vi "Excel input(SubVI).vi"(8 "error in (no error)":errorcluster, 11 "The Path to save excel":path=path "E:/程序完善/油菜/side_features") -> (0 "error out":errorcluster, 3 "Cluster":T1)   [LabVIEW 2015]
uses:
  <vilib>/Utility/NIReport.llb/NI_report.lvclass
  <vilib>/addons/_office/_exclsub.llb/font.ctl
  <vilib>/addons/_office/NI_ReportGenerationToolkit.lvlib
  <vilib>/Utility/NIReport.llb/Excel/NI_Excel.lvclass
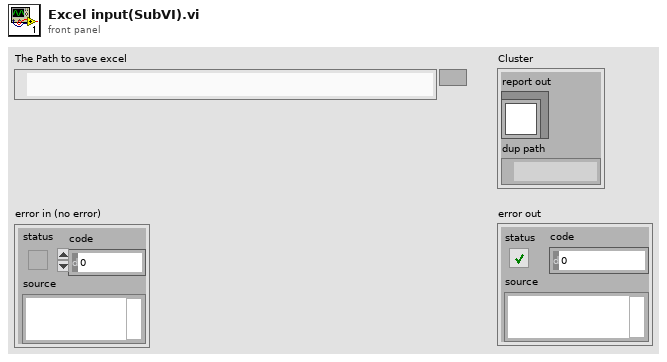
[diagram p1: front panel]
types:
  T1 = cluster{"report out":refnum<class "NI_report.lvclass">, "dup path":path}
  T2 = enum16{"maximized", "minimized", "normal", "no change"}
  T3 = typedef "NI_ReportGenerationToolkit.lvlib/font.ctl" = cluster{"font name":string, "font size":dbl, "bold":u16, "italic":u16, "underline":u16, "strike through":u16, "font color":u32}
  T4 = enum16{"Standard Report", "HTML", "Word", "Excel"}
diagram:
  w408 = T3 {"font name"="", "font size"=13.0, "bold"=0, "italic"=0, "underline"=0, "strike through"=0, "font color"=16777216} ("font")
  w106 = 0 ("column")
  n1 = call <vilib>:"New Report.vi"("window state (normal)"=T2."normal", "report type"=T4."Excel", "error in (no error)"="error in (no error)") -> ("report out"=w10:refnum<class "NI_report.lvclass">, "error out"=w7:errorcluster)  [unwired: 3 in, 8 out]
  n2 = call <vilib>:"Excel Easy Title.vi"("report in"=w10, "title"="Side Features", "start (0, 0)"=cluster{"row":i32, "column":i32} {"row"=0, "column"=0}, "font"=T3 {"font name"="", "font size"=16.0, "bold"=1, "italic"=2, "underline"=2, "strike through"=2, "font color"=0}, "error in (no error)"=w7) -> ("report out"=w107:refnum<class "NI_report.lvclass">, "error out"=w110:errorcluster)  [unwired: 1 in, 8 out]
  n3 = Bundle("row"=1, "column"=w106) -> (w109:cluster{"row":i32, "column":i32})  [unwired: 1 out]
  n4 = Increment(x=w106) -> (x+1=w45:i32)
  n5 = call <vilib>:"Excel Easy Text.vi"("report in"=w107, "border? (F)"=FALSE, "font"=w408, "text"="Serial number", "start (-1, -1)"=w109, "error in (no error)"=w110) -> ("report out"=w56:refnum<class "NI_report.lvclass">, "error out"=w43:errorcluster)  [unwired: 2 in, 6 out]
  n6 = Bundle("row"=1, w45) -> (w60:cluster{"row":i32, i32})  [unwired: 1 out]
  n7 = Increment(x=w45) -> (x+1=w44:i32)
  n8 = call <vilib>:"Excel Easy Text.vi"("report in"=w56, "border? (F)"=FALSE, "font"=w408, "text"="M_TEX_SV", "start (-1, -1)"=w60, "error in (no error)"=w43) -> ("report out"=w47:refnum<class "NI_report.lvclass">, "error out"=w42:errorcluster)  [unwired: 2 in, 6 out]
  n9 = Bundle("row"=1, w44) -> (w52:cluster{"row":i32, i32})  [unwired: 1 out]
  n10 = Increment(x=w44) -> (x+1=w20:i32)
  n11 = call <vilib>:"Excel Easy Text.vi"("report in"=w47, "border? (F)"=FALSE, "font"=w408, "text"="SE_TEX_SV", "start (-1, -1)"=w52, "error in (no error)"=w42) -> ("report out"=w46:refnum<class "NI_report.lvclass">, "error out"=w41:errorcluster)  [unwired: 2 in, 6 out]
  n12 = Bundle("row"=1, w20) -> (w51:cluster{"row":i32, i32})  [unwired: 1 out]
  n13 = Increment(x=w20) -> (x+1=w26:i32)
  n14 = call <vilib>:"Excel Easy Text.vi"("report in"=w46, "border? (F)"=FALSE, "font"=w408, "text"="S_TEX_SV", "start (-1, -1)"=w51, "error in (no error)"=w41) -> ("report out"=w21:refnum<class "NI_report.lvclass">, "error out"=w22:errorcluster)  [unwired: 2 in, 6 out]
  n15 = Bundle("row"=1, w26) -> (w40:cluster{"row":i32, i32})  [unwired: 1 out]
  n16 = Increment(x=w26) -> (x+1=w25:i32)
  n17 = call <vilib>:"Excel Easy Text.vi"("report in"=w21, "border? (F)"=FALSE, "font"=w408, "text"="MU3_TEX_SV", "start (-1, -1)"=w40, "error in (no error)"=w22) -> ("report out"=w28:refnum<class "NI_report.lvclass">, "error out"=w24:errorcluster)  [unwired: 2 in, 6 out]
  n18 = Bundle("row"=1, w25) -> (w33:cluster{"row":i32, i32})  [unwired: 1 out]
  n19 = Increment(x=w25) -> (x+1=w13:i32)
  n20 = call <vilib>:"Excel Easy Text.vi"("report in"=w28, "border? (F)"=FALSE, "font"=w408, "text"="U_TEX_SV", "start (-1, -1)"=w33, "error in (no error)"=w24) -> ("report out"=w27:refnum<class "NI_report.lvclass">, "error out"=w23:errorcluster)  [unwired: 2 in, 6 out]
  n21 = Bundle("row"=1, w13) -> (w32:cluster{"row":i32, i32})  [unwired: 1 out]
  n22 = Increment(x=w13) -> (x+1=w75:i32)
  n23 = call <vilib>:"Excel Easy Text.vi"("report in"=w27, "border? (F)"=FALSE, "font"=w408, "text"="E_TEX_SV", "start (-1, -1)"=w32, "error in (no error)"=w23) -> ("report out"=w15:refnum<class "NI_report.lvclass">, "error out"=w14:errorcluster)  [unwired: 2 in, 6 out]
  n24 = Bundle("row"=1, w75) -> (w16:cluster{"row":i32, i32})  [unwired: 1 out]
  n25 = Increment(x=w75) -> (x+1=w78:i32)
  n26 = call <vilib>:"Excel Easy Text.vi"("report in"=w15, "border? (F)"=FALSE, "font"=w408, "text"="TPA_SV", "start (-1, -1)"=w16, "error in (no error)"=w14) -> ("report out"=w73:refnum<class "NI_report.lvclass">, "error out"=w74:errorcluster)  [unwired: 2 in, 6 out]
  n27 = Bundle("row"=1, w78) -> (w69:cluster{"row":i32, i32})  [unwired: 1 out]
  n28 = Increment(x=w78) -> (x+1=w81:i32)
  n29 = call <vilib>:"Excel Easy Text.vi"("report in"=w73, "border? (F)"=FALSE, "font"=w408, "text"="H_SV", "start (-1, -1)"=w69, "error in (no error)"=w74) -> ("report out"=w76:refnum<class "NI_report.lvclass">, "error out"=w77:errorcluster)  [unwired: 2 in, 6 out]
  n30 = Bundle("row"=1, w81) -> (w61:cluster{"row":i32, i32})  [unwired: 1 out]
  n31 = Increment(x=w81) -> (x+1=w88:i32)
  n32 = call <vilib>:"Excel Easy Text.vi"("report in"=w76, "border? (F)"=FALSE, "font"=w408, "text"="W_SV", "start (-1, -1)"=w61, "error in (no error)"=w77) -> ("report out"=w79:refnum<class "NI_report.lvclass">, "error out"=w80:errorcluster)  [unwired: 2 in, 6 out]
  n33 = Bundle("row"=1, w88) -> (w65:cluster{"row":i32, i32})  [unwired: 1 out]
  n34 = Increment(x=w88) -> (x+1=w95:i32)
  n35 = call <vilib>:"Excel Easy Text.vi"("report in"=w79, "border? (F)"=FALSE, "font"=w408, "text"="HWR_SV", "start (-1, -1)"=w65, "error in (no error)"=w80) -> ("report out"=w86:refnum<class "NI_report.lvclass">, "error out"=w87:errorcluster)  [unwired: 2 in, 6 out]
  n36 = Bundle("row"=1, w95) -> (w82:cluster{"row":i32, i32})  [unwired: 1 out]
  n37 = Increment(x=w95) -> (x+1=w102:i32)
  n38 = call <vilib>:"Excel Easy Text.vi"("report in"=w86, "border? (F)"=FALSE, "font"=w408, "text"="FDNIC_SV", "start (-1, -1)"=w82, "error in (no error)"=w87) -> ("report out"=w93:refnum<class "NI_report.lvclass">, "error out"=w94:errorcluster)  [unwired: 2 in, 6 out]
  n39 = Bundle("row"=1, w102) -> (w89:cluster{"row":i32, i32})  [unwired: 1 out]
  n40 = Increment(x=w102) -> (x+1=w104:i32)
  n41 = call <vilib>:"Excel Easy Text.vi"("report in"=w93, "border? (F)"=FALSE, "font"=w408, "text"="FDIC_SV", "start (-1, -1)"=w89, "error in (no error)"=w94) -> ("report out"=w100:refnum<class "NI_report.lvclass">, "error out"=w101:errorcluster)  [unwired: 2 in, 6 out]
  n42 = Bundle("row"=1, w104) -> (w96:cluster{"row":i32, i32})  [unwired: 1 out]
  n43 = Increment(x=w104) -> (x+1=w151:i32)
  n44 = call <vilib>:"Excel Easy Text.vi"("report in"=w100, "border? (F)"=FALSE, "font"=w408, "text"="R_SV", "start (-1, -1)"=w96, "error in (no error)"=w101) -> ("report out"=w150:refnum<class "NI_report.lvclass">, "error out"=w152:errorcluster)  [unwired: 2 in, 6 out]
  n45 = Bundle("row"=1, w151) -> (w149:cluster{"row":i32, i32})  [unwired: 1 out]
  n46 = Increment(x=w151) -> (x+1=w125:i32)
  n47 = call <vilib>:"Excel Easy Text.vi"("report in"=w150, "border? (F)"=FALSE, "font"=w408, "text"="PAR_SV", "start (-1, -1)"=w149, "error in (no error)"=w152) -> ("report out"=w121:refnum<class "NI_report.lvclass">, "error out"=w122:errorcluster)  [unwired: 2 in, 6 out]
  n48 = Bundle("row"=1, w125) -> (w111:cluster{"row":i32, i32})  [unwired: 1 out]
  n49 = Increment(x=w125) -> (x+1=w132:i32)
  n50 = call <vilib>:"Excel Easy Text.vi"("report in"=w121, "border? (F)"=FALSE, "font"=w408, "text"="HA_SV", "start (-1, -1)"=w111, "error in (no error)"=w122) -> ("report out"=w123:refnum<class "NI_report.lvclass">, "error out"=w124:errorcluster)  [unwired: 2 in, 6 out]
  n51 = Bundle("row"=1, w132) -> (w115:cluster{"row":i32, i32})  [unwired: 1 out]
  n52 = Increment(x=w132) -> (x+1=w139:i32)
  n53 = call <vilib>:"Excel Easy Text.vi"("report in"=w123, "border? (F)"=FALSE, "font"=w408, "text"="AC_SV", "start (-1, -1)"=w115, "error in (no error)"=w124) -> ("report out"=w130:refnum<class "NI_report.lvclass">, "error out"=w131:errorcluster)  [unwired: 2 in, 6 out]
  n54 = Bundle("row"=1, w139) -> (w126:cluster{"row":i32, i32})  [unwired: 1 out]
  n55 = Increment(x=w139) -> (x+1=w146:i32)
  n56 = call <vilib>:"Excel Easy Text.vi"("report in"=w130, "border? (F)"=FALSE, "font"=w408, "text"="M_TEX_SV_FL", "start (-1, -1)"=w126, "error in (no error)"=w131) -> ("report out"=w137:refnum<class "NI_report.lvclass">, "error out"=w138:errorcluster)  [unwired: 2 in, 6 out]
  n57 = Bundle("row"=1, w146) -> (w133:cluster{"row":i32, i32})  [unwired: 1 out]
  n58 = Increment(x=w146) -> (x+1=w148:i32)
  n59 = call <vilib>:"Excel Easy Text.vi"("report in"=w137, "border? (F)"=FALSE, "font"=w408, "text"="SE_TEX_SV_FL", "start (-1, -1)"=w133, "error in (no error)"=w138) -> ("report out"=w144:refnum<class "NI_report.lvclass">, "error out"=w145:errorcluster)  [unwired: 2 in, 6 out]
  n60 = Bundle("row"=1, w148) -> (w140:cluster{"row":i32, i32})  [unwired: 1 out]
  n61 = Increment(x=w148) -> (x+1=w219:i32)
  n62 = call <vilib>:"Excel Easy Text.vi"("report in"=w144, "border? (F)"=FALSE, "font"=w408, "text"="S_TEX_SV_FL", "start (-1, -1)"=w140, "error in (no error)"=w145) -> ("report out"=w221:refnum<class "NI_report.lvclass">, "error out"=w222:errorcluster)  [unwired: 2 in, 6 out]
  n63 = Bundle("row"=1, w219) -> (w220:cluster{"row":i32, i32})  [unwired: 1 out]
  n64 = Increment(x=w219) -> (x+1=w167:i32)
  n65 = call <vilib>:"Excel Easy Text.vi"("report in"=w221, "border? (F)"=FALSE, "font"=w408, "text"="MU3_TEX_SV_FL", "start (-1, -1)"=w220, "error in (no error)"=w222) -> ("report out"=w159:refnum<class "NI_report.lvclass">, "error out"=w160:errorcluster)  [unwired: 2 in, 6 out]
  n66 = Bundle("row"=1, w167) -> (w155:cluster{"row":i32, i32})  [unwired: 1 out]
  n67 = Increment(x=w167) -> (x+1=w174:i32)
  n68 = call <vilib>:"Excel Easy Text.vi"("report in"=w159, "border? (F)"=FALSE, "font"=w408, "text"="U_TEX_SV_FL", "start (-1, -1)"=w155, "error in (no error)"=w160) -> ("report out"=w165:refnum<class "NI_report.lvclass">, "error out"=w166:errorcluster)  [unwired: 2 in, 6 out]
  n69 = Bundle("row"=1, w174) -> (w161:cluster{"row":i32, i32})  [unwired: 1 out]
  n70 = Increment(x=w174) -> (x+1=w176:i32)
  n71 = call <vilib>:"Excel Easy Text.vi"("report in"=w165, "border? (F)"=FALSE, "font"=w408, "text"="E_TEX_SV_FL", "start (-1, -1)"=w161, "error in (no error)"=w166) -> ("report out"=w172:refnum<class "NI_report.lvclass">, "error out"=w173:errorcluster)  [unwired: 2 in, 6 out]
  n72 = Bundle("row"=1, w176) -> (w168:cluster{"row":i32, i32})  [unwired: 1 out]
  n73 = Increment(x=w176) -> (x+1=w217:i32)
  n74 = call <vilib>:"Excel Easy Text.vi"("report in"=w172, "border? (F)"=FALSE, "font"=w408, "text"="YPA_SV_FL", "start (-1, -1)"=w168, "error in (no error)"=w173) -> ("report out"=w216:refnum<class "NI_report.lvclass">, "error out"=w218:errorcluster)  [unwired: 2 in, 6 out]
  n75 = Bundle("row"=1, w217) -> (w215:cluster{"row":i32, i32})  [unwired: 1 out]
  n76 = Increment(x=w217) -> (x+1=w191:i32)
  n77 = call <vilib>:"Excel Easy Text.vi"("report in"=w216, "border? (F)"=FALSE, "font"=w408, "text"="H_SV_FL", "start (-1, -1)"=w215, "error in (no error)"=w218) -> ("report out"=w187:refnum<class "NI_report.lvclass">, "error out"=w188:errorcluster)  [unwired: 2 in, 6 out]
  n78 = Bundle("row"=1, w191) -> (w177:cluster{"row":i32, i32})  [unwired: 1 out]
  n79 = Increment(x=w191) -> (x+1=w198:i32)
  n80 = call <vilib>:"Excel Easy Text.vi"("report in"=w187, "border? (F)"=FALSE, "font"=w408, "text"="W_SV_FL", "start (-1, -1)"=w177, "error in (no error)"=w188) -> ("report out"=w189:refnum<class "NI_report.lvclass">, "error out"=w190:errorcluster)  [unwired: 2 in, 6 out]
  n81 = Bundle("row"=1, w198) -> (w181:cluster{"row":i32, i32})  [unwired: 1 out]
  n82 = Increment(x=w198) -> (x+1=w205:i32)
  n83 = call <vilib>:"Excel Easy Text.vi"("report in"=w189, "border? (F)"=FALSE, "font"=w408, "text"="HWR_SV_FL", "start (-1, -1)"=w181, "error in (no error)"=w190) -> ("report out"=w196:refnum<class "NI_report.lvclass">, "error out"=w197:errorcluster)  [unwired: 2 in, 6 out]
  n84 = Bundle("row"=1, w205) -> (w192:cluster{"row":i32, i32})  [unwired: 1 out]
  n85 = Increment(x=w205) -> (x+1=w212:i32)
  n86 = call <vilib>:"Excel Easy Text.vi"("report in"=w196, "border? (F)"=FALSE, "font"=w408, "text"="FDNIC_SV_FL", "start (-1, -1)"=w192, "error in (no error)"=w197) -> ("report out"=w203:refnum<class "NI_report.lvclass">, "error out"=w204:errorcluster)  [unwired: 2 in, 6 out]
  n87 = Bundle("row"=1, w212) -> (w199:cluster{"row":i32, i32})  [unwired: 1 out]
  n88 = Increment(x=w212) -> (x+1=w214:i32)
  n89 = call <vilib>:"Excel Easy Text.vi"("report in"=w203, "border? (F)"=FALSE, "font"=w408, "text"="FDIC_SV_FL", "start (-1, -1)"=w199, "error in (no error)"=w204) -> ("report out"=w210:refnum<class "NI_report.lvclass">, "error out"=w211:errorcluster)  [unwired: 2 in, 6 out]
  n90 = Bundle("row"=1, w214) -> (w206:cluster{"row":i32, i32})  [unwired: 1 out]
  n91 = Increment(x=w214) -> (x+1=w338:i32)
  n92 = call <vilib>:"Excel Easy Text.vi"("report in"=w210, "border? (F)"=FALSE, "font"=w408, "text"="R_SV_FL", "start (-1, -1)"=w206, "error in (no error)"=w211) -> ("report out"=w339:refnum<class "NI_report.lvclass">, "error out"=w340:errorcluster)  [unwired: 2 in, 6 out]
  n93 = Bundle("row"=1, w338) -> (w341:cluster{"row":i32, i32})  [unwired: 1 out]
  n94 = Increment(x=w338) -> (x+1=w266:i32)
  n95 = call <vilib>:"Excel Easy Text.vi"("report in"=w339, "border? (F)"=FALSE, "font"=w408, "text"="PAR_SV_FL", "start (-1, -1)"=w341, "error in (no error)"=w340) -> ("report out"=w265:refnum<class "NI_report.lvclass">, "error out"=w267:errorcluster)  [unwired: 2 in, 6 out]
  n96 = Bundle("row"=1, w266) -> (w264:cluster{"row":i32, i32})  [unwired: 1 out]
  n97 = Increment(x=w266) -> (x+1=w240:i32)
  n98 = call <vilib>:"Excel Easy Text.vi"("report in"=w265, "border? (F)"=FALSE, "font"=w408, "text"="HA_SV_FL", "start (-1, -1)"=w264, "error in (no error)"=w267) -> ("report out"=w236:refnum<class "NI_report.lvclass">, "error out"=w237:errorcluster)  [unwired: 2 in, 6 out]
  n99 = Bundle("row"=1, w240) -> (w226:cluster{"row":i32, i32})  [unwired: 1 out]
  n100 = Increment(x=w240) -> (x+1=w247:i32)
  n101 = call <vilib>:"Excel Easy Text.vi"("report in"=w236, "border? (F)"=FALSE, "font"=w408, "text"="AC_SV_FL", "start (-1, -1)"=w226, "error in (no error)"=w237) -> ("report out"=w238:refnum<class "NI_report.lvclass">, "error out"=w239:errorcluster)  [unwired: 2 in, 6 out]
  n102 = Bundle("row"=1, w247) -> (w230:cluster{"row":i32, i32})  [unwired: 1 out]
  n103 = Increment(x=w247) -> (x+1=w254:i32)
  n104 = call <vilib>:"Excel Easy Text.vi"("report in"=w238, "border? (F)"=FALSE, "font"=w408, "text"="FN_SV", "start (-1, -1)"=w230, "error in (no error)"=w239) -> ("report out"=w245:refnum<class "NI_report.lvclass">, "error out"=w246:errorcluster)  [unwired: 2 in, 6 out]
  n105 = Bundle("row"=1, w254) -> (w241:cluster{"row":i32, i32})  [unwired: 1 out]
  n106 = Increment(x=w254) -> (x+1=w261:i32)
  n107 = call <vilib>:"Excel Easy Text.vi"("report in"=w245, "border? (F)"=FALSE, "font"=w408, "text"="GPA_SV", "start (-1, -1)"=w241, "error in (no error)"=w246) -> ("report out"=w252:refnum<class "NI_report.lvclass">, "error out"=w253:errorcluster)  [unwired: 2 in, 6 out]
  n108 = Bundle("row"=1, w261) -> (w248:cluster{"row":i32, i32})  [unwired: 1 out]
  n109 = Increment(x=w261) -> (x+1=w263:i32)
  n110 = call <vilib>:"Excel Easy Text.vi"("report in"=w252, "border? (F)"=FALSE, "font"=w408, "text"="GPAR_SV", "start (-1, -1)"=w248, "error in (no error)"=w253) -> ("report out"=w259:refnum<class "NI_report.lvclass">, "error out"=w260:errorcluster)  [unwired: 2 in, 6 out]
  n111 = Bundle("row"=1, w263) -> (w255:cluster{"row":i32, i32})  [unwired: 1 out]
  n112 = Increment(x=w263) -> (x+1=w334:i32)
  n113 = call <vilib>:"Excel Easy Text.vi"("report in"=w259, "border? (F)"=FALSE, "font"=w408, "text"="YPAR_SV", "start (-1, -1)"=w255, "error in (no error)"=w260) -> ("report out"=w336:refnum<class "NI_report.lvclass">, "error out"=w337:errorcluster)  [unwired: 2 in, 6 out]
  n114 = Bundle("row"=1, w334) -> (w335:cluster{"row":i32, i32})  [unwired: 1 out]
  n115 = Increment(x=w334) -> (x+1=w282:i32)
  n116 = call <vilib>:"Excel Easy Text.vi"("report in"=w336, "border? (F)"=FALSE, "font"=w408, "text"="PC1_SV", "start (-1, -1)"=w335, "error in (no error)"=w337) -> ("report out"=w274:refnum<class "NI_report.lvclass">, "error out"=w275:errorcluster)  [unwired: 2 in, 6 out]
  n117 = Bundle("row"=1, w282) -> (w270:cluster{"row":i32, i32})  [unwired: 1 out]
  n118 = Increment(x=w282) -> (x+1=w289:i32)
  n119 = call <vilib>:"Excel Easy Text.vi"("report in"=w274, "border? (F)"=FALSE, "font"=w408, "text"="PC2_SV", "start (-1, -1)"=w270, "error in (no error)"=w275) -> ("report out"=w280:refnum<class "NI_report.lvclass">, "error out"=w281:errorcluster)  [unwired: 2 in, 6 out]
  n120 = Bundle("row"=1, w289) -> (w276:cluster{"row":i32, i32})  [unwired: 1 out]
  n121 = Increment(x=w289) -> (x+1=w291:i32)
  n122 = call <vilib>:"Excel Easy Text.vi"("report in"=w280, "border? (F)"=FALSE, "font"=w408, "text"="PC3_SV", "start (-1, -1)"=w276, "error in (no error)"=w281) -> ("report out"=w287:refnum<class "NI_report.lvclass">, "error out"=w288:errorcluster)  [unwired: 2 in, 6 out]
  n123 = Bundle("row"=1, w291) -> (w283:cluster{"row":i32, i32})  [unwired: 1 out]
  n124 = Increment(x=w291) -> (x+1=w332:i32)
  n125 = call <vilib>:"Excel Easy Text.vi"("report in"=w287, "border? (F)"=FALSE, "font"=w408, "text"="PC4_SV", "start (-1, -1)"=w283, "error in (no error)"=w288) -> ("report out"=w331:refnum<class "NI_report.lvclass">, "error out"=w333:errorcluster)  [unwired: 2 in, 6 out]
  n126 = Bundle("row"=1, w332) -> (w330:cluster{"row":i32, i32})  [unwired: 1 out]
  n127 = Increment(x=w332) -> (x+1=w306:i32)
  n128 = call <vilib>:"Excel Easy Text.vi"("report in"=w331, "border? (F)"=FALSE, "font"=w408, "text"="PC5_SV", "start (-1, -1)"=w330, "error in (no error)"=w333) -> ("report out"=w302:refnum<class "NI_report.lvclass">, "error out"=w303:errorcluster)  [unwired: 2 in, 6 out]
  n129 = Bundle("row"=1, w306) -> (w292:cluster{"row":i32, i32})  [unwired: 1 out]
  n130 = Increment(x=w306) -> (x+1=w313:i32)
  n131 = call <vilib>:"Excel Easy Text.vi"("report in"=w302, "border? (F)"=FALSE, "font"=w408, "text"="PC6_SV", "start (-1, -1)"=w292, "error in (no error)"=w303) -> ("report out"=w304:refnum<class "NI_report.lvclass">, "error out"=w305:errorcluster)  [unwired: 2 in, 6 out]
  n132 = Bundle("row"=1, w313) -> (w296:cluster{"row":i32, i32})  [unwired: 1 out]
  n133 = Increment(x=w313) -> (x+1=w320:i32)
  n134 = call <vilib>:"Excel Easy Text.vi"("report in"=w304, "border? (F)"=FALSE, "font"=w408, "text"="F1", "start (-1, -1)"=w296, "error in (no error)"=w305) -> ("report out"=w311:refnum<class "NI_report.lvclass">, "error out"=w312:errorcluster)  [unwired: 2 in, 6 out]
  n135 = Bundle("row"=1, w320) -> (w307:cluster{"row":i32, i32})  [unwired: 1 out]
  n136 = Increment(x=w320) -> (x+1=w327:i32)
  n137 = call <vilib>:"Excel Easy Text.vi"("report in"=w311, "border? (F)"=FALSE, "font"=w408, "text"="F2", "start (-1, -1)"=w307, "error in (no error)"=w312) -> ("report out"=w318:refnum<class "NI_report.lvclass">, "error out"=w319:errorcluster)  [unwired: 2 in, 6 out]
  n138 = Bundle("row"=1, w327) -> (w314:cluster{"row":i32, i32})  [unwired: 1 out]
  n139 = Increment(x=w327) -> (x+1=w329:i32)
  n140 = call <vilib>:"Excel Easy Text.vi"("report in"=w318, "border? (F)"=FALSE, "font"=w408, "text"="F3", "start (-1, -1)"=w314, "error in (no error)"=w319) -> ("report out"=w325:refnum<class "NI_report.lvclass">, "error out"=w326:errorcluster)  [unwired: 2 in, 6 out]
  n141 = Bundle("row"=1, w329) -> (w321:cluster{"row":i32, i32})  [unwired: 1 out]
  n142 = Increment(x=w329) -> (x+1=w411:i32)
  n143 = call <vilib>:"Excel Easy Text.vi"("report in"=w325, "border? (F)"=FALSE, "font"=w408, "text"="F4", "start (-1, -1)"=w321, "error in (no error)"=w326) -> ("report out"=w410:refnum<class "NI_report.lvclass">, "error out"=w407:errorcluster)  [unwired: 2 in, 6 out]
  n144 = Bundle("row"=1, w411) -> (w409:cluster{"row":i32, i32})  [unwired: 1 out]
  n145 = Increment(x=w411) -> (x+1=w351:i32)
  n146 = call <vilib>:"Excel Easy Text.vi"("report in"=w410, "border? (F)"=FALSE, "font"=w408, "text"="F5", "start (-1, -1)"=w409, "error in (no error)"=w407) -> ("report out"=w348:refnum<class "NI_report.lvclass">, "error out"=w349:errorcluster)  [unwired: 2 in, 6 out]
  n147 = Bundle("row"=1, w351) -> (w344:cluster{"row":i32, i32})  [unwired: 1 out]
  n148 = Increment(x=w351) -> (x+1=w403:i32)
  n149 = call <vilib>:"Excel Easy Text.vi"("report in"=w348, "border? (F)"=FALSE, "font"=w408, "text"="F6", "start (-1, -1)"=w344, "error in (no error)"=w349) -> ("report out"=w405:refnum<class "NI_report.lvclass">, "error out"=w406:errorcluster)  [unwired: 2 in, 6 out]
  n150 = Bundle("row"=1, w403) -> (w404:cluster{"row":i32, i32})  [unwired: 1 out]
  n151 = Increment(x=w403) -> (x+1=w366:i32)
  n152 = call <vilib>:"Excel Easy Text.vi"("report in"=w405, "border? (F)"=FALSE, "font"=w408, "text"="F7", "start (-1, -1)"=w404, "error in (no error)"=w406) -> ("report out"=w358:refnum<class "NI_report.lvclass">, "error out"=w359:errorcluster)  [unwired: 2 in, 6 out]
  n153 = Bundle("row"=1, w366) -> (w354:cluster{"row":i32, i32})  [unwired: 1 out]
  n154 = Increment(x=w366) -> (x+1=w373:i32)
  n155 = call <vilib>:"Excel Easy Text.vi"("report in"=w358, "border? (F)"=FALSE, "font"=w408, "text"="F8", "start (-1, -1)"=w354, "error in (no error)"=w359) -> ("report out"=w364:refnum<class "NI_report.lvclass">, "error out"=w365:errorcluster)  [unwired: 2 in, 6 out]
  n156 = Bundle("row"=1, w373) -> (w360:cluster{"row":i32, i32})  [unwired: 1 out]
  n157 = Increment(x=w373) -> (x+1=w375:i32)
  n158 = call <vilib>:"Excel Easy Text.vi"("report in"=w364, "border? (F)"=FALSE, "font"=w408, "text"="F9", "start (-1, -1)"=w360, "error in (no error)"=w365) -> ("report out"=w371:refnum<class "NI_report.lvclass">, "error out"=w372:errorcluster)  [unwired: 2 in, 6 out]
  n159 = Bundle("row"=1, w375) -> (w367:cluster{"row":i32, i32})  [unwired: 1 out]
  n160 = Increment(x=w375) -> (x+1=w401:i32)
  n161 = call <vilib>:"Excel Easy Text.vi"("report in"=w371, "border? (F)"=FALSE, "font"=w408, "text"="F10", "start (-1, -1)"=w367, "error in (no error)"=w372) -> ("report out"=w400:refnum<class "NI_report.lvclass">, "error out"=w402:errorcluster)  [unwired: 2 in, 6 out]
  n162 = Bundle("row"=1, w401) -> (w399:cluster{"row":i32, i32})  [unwired: 1 out]
  n163 = call <vilib>:"Check if File or Folder Exists.vi"("path"="The Path to save excel") -> ("error out"=w419:errorcluster, "file or folder exists?"=w417:bool, "dup path"=w418:path)  [unwired: 8 in]
  n164 = Increment(x=w401) -> (x+1=w390:i32)
  n165 = case shown="True" w417 {
    tunnel: [w424 w429] -> w2
    tunnel: w418 -> [w424 w425]
    tunnel: w419 -> [_ _]
    frame False {
    }
    frame True {
      n166 = Get Date/Time In Seconds() -> (seconds since 1Jan1904=w431:timestamp)
      n167 = Path To String(path=w425) -> (string=w428:string)
      n168 = Format Date/Time String(time format string (%c)="side_features.xls", seconds (now)=w431) -> (date/time string=w427:string)  [unwired: 1 out]
      n169 = Concatenate Strings(w428, w427) -> (w426:string)
      n170 = String To Path(string=w426) -> (path=w429:path)
    }
  }
  n171 = call <vilib>:"Excel Easy Text.vi"("report in"=w400, "border? (F)"=FALSE, "font"=w408, "text"="F11", "start (-1, -1)"=w399, "error in (no error)"=w402) -> ("report out"=w386:refnum<class "NI_report.lvclass">, "error out"=w387:errorcluster)  [unwired: 2 in, 6 out]
  n172 = Bundle("row"=1, w390) -> (w376:cluster{"row":i32, i32})  [unwired: 1 out]
  n173 = Increment(x=w390) -> (x+1=w397:i32)
  n174 = call <vilib>:"Excel Easy Text.vi"("report in"=w386, "border? (F)"=FALSE, "font"=w408, "text"="F12", "start (-1, -1)"=w376, "error in (no error)"=w387) -> ("report out"=w388:refnum<class "NI_report.lvclass">, "error out"=w389:errorcluster)  [unwired: 2 in, 6 out]
  n175 = Bundle("row"=1, w397) -> (w380:cluster{"row":i32, i32})  [unwired: 1 out]
  n176 = Increment(x=w397) -> (x+1=w398:i32)
  n177 = call <vilib>:"Excel Easy Text.vi"("report in"=w388, "border? (F)"=FALSE, "font"=w408, "text"="F13", "start (-1, -1)"=w380, "error in (no error)"=w389) -> ("report out"=w395:refnum<class "NI_report.lvclass">, "error out"=w396:errorcluster)  [unwired: 2 in, 6 out]
  n178 = Bundle("row"=1, w398) -> (w391:cluster{"row":i32, i32})  [unwired: 1 out]
  n179 = call <vilib>:"Excel Easy Text.vi"("report in"=w395, "border? (F)"=FALSE, "font"=w408, "text"="F14", "start (-1, -1)"=w391, "error in (no error)"=w396) -> ("report out"=w412:refnum<class "NI_report.lvclass">, "error out"=w413:errorcluster)  [unwired: 2 in, 6 out]
  n180 = call <vilib>:"Excel Set Cell Dimension.vi"("report in"=w412, "width (-1)"=1.2, "error in (no error)"=w413) -> ("report out"=w414:refnum<class "NI_report.lvclass">, "error out"=w415:errorcluster)  [unwired: 11 in]
  n181 = call <vilib>:"Excel Get ActiveX References.vi"("report in"=w414, "error in (no error)"=w415) -> ("report out"=w420:refnum<class "NI_report.lvclass">, "Excel._Workbook"=w4:refnum<k7>, "error out"=w3:errorcluster)  [unwired: 7 in, 4 out]
  n182 = invoke class="_Workbook" method="SaveAs"(reference=w4, error in=w3, "Filename"=w2) -> (error out=→"error out":errorcluster)  [unwired: 13 in, 15 out]
  n183 = Bundle("report out"=w420, "dup path"=w2) -> (→"Cluster":T1)  [unwired: 1 in]
